vi "Write Terminal Size.vi"(8 "Error In":errorcluster, 10 "Size":cluster{"Width":i32, "Height":i32}, 11 "Channel In":refnum<class "Channel.lvclass">) -> (0 "Error Out":errorcluster, 3 "Channel Out":refnum<class "Channel.lvclass">)   [LabVIEW 2018, in "Toolkit.lvlib" / "Channel.lvclass"]
uses:
  Channel.lvclass
  Channel.lvclass/Channel.ctl
  Session/Session.lvclass/Session.ctl
  SSH/SSH.lvclass/SSH.ctl
  Session/Session.lvclass
  Toolkit.lvlib
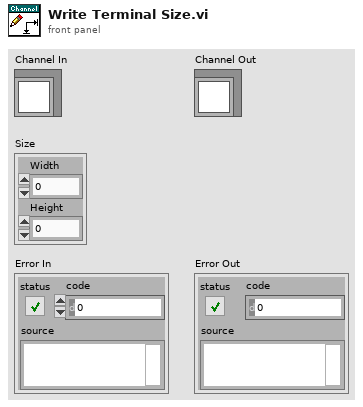
[diagram p1: front panel]
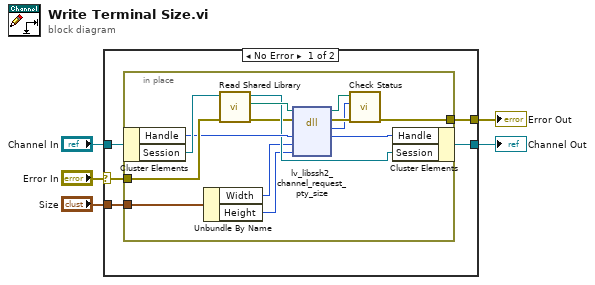
[diagram p0: block diagram]
diagram:
  n1 = case shown="No Error" "Error In" {
    selector: "Error In" -> [w8 w26]
    tunnel: [w7 w26] -> w4
    tunnel: "Channel In" -> [w10 w25]
    tunnel: [w9 w25] -> w2
    tunnel: "Size" -> [w6 _]
    frame No Error {
      n2 = in-place {
        in-place-border: w8 -> [w22]
        in-place-border: [w18] -> w7
        in-place-border: w6 -> [w13]
        n3 = in-place-cluster #1(w10) -> ("Handle"=w17:u64, "Session"=w24:refnum<class "Session.lvclass">)
        n4 = Unbundle By Name(w13) -> ("Width"=w12:i32, "Height"=w11:i32)
        n5 = call "Read Shared Library.vi"("Error In"=w22, "Session In"=w24) -> ("Erorr Out"=w14:errorcluster, "libssh2lv Shared Library"=w23:path, "Session Out"=w15:refnum<class "Session.lvclass">)  [unwired: 7 in]
        n6 = dll-call lib="libssh2lv.*" fn="lv_libssh2_channel_request_pty_size"(path in=w23, error in=w14, "handle"=w17, "width"=w12, "height"=w11) -> (path out=w20:path, error out=w21:errorcluster, "status"=w19:i32, "handle"=w16:u64)  [unwired: 3 in]
        n7 = call "Check Status.vi"("Error In"=w21, "Status"=w19, "lv-libssh2 Shared Library In"=w20) -> ("Error Out"=w18:errorcluster)  [unwired: 7 in, 1 out]
        n8 = in-place-cluster #1("Handle"=w16, "Session"=w15) -> (w9:refnum<class "Channel.lvclass">)
      }
    }
    frame Error {
    }
  }
  "Error Out" <- w4
  "Channel Out" <- w2
